vi "fo_SaveDatasetToFile.vi"(8 "error in (no error)":errorcluster, 9 "patientID":string="HALLO", 10 "Dataset index":i32, 11 "Results":refnum<k24>) -> (0 "error out":errorcluster)   [LabVIEW 2013, in "main.lvlib"]
uses:
  main.lvlib
  C:/Users/Simon/SkyDrive/LabView/2013/DM2020/bin/Dicom.dll
  bin/Dicom.dll
  Globals/DataPathGlobalVariable.vi
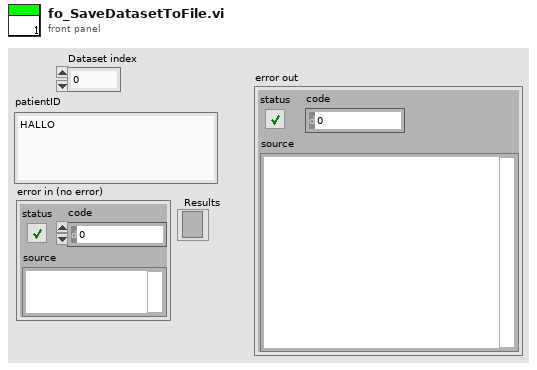
[diagram p1: front panel]
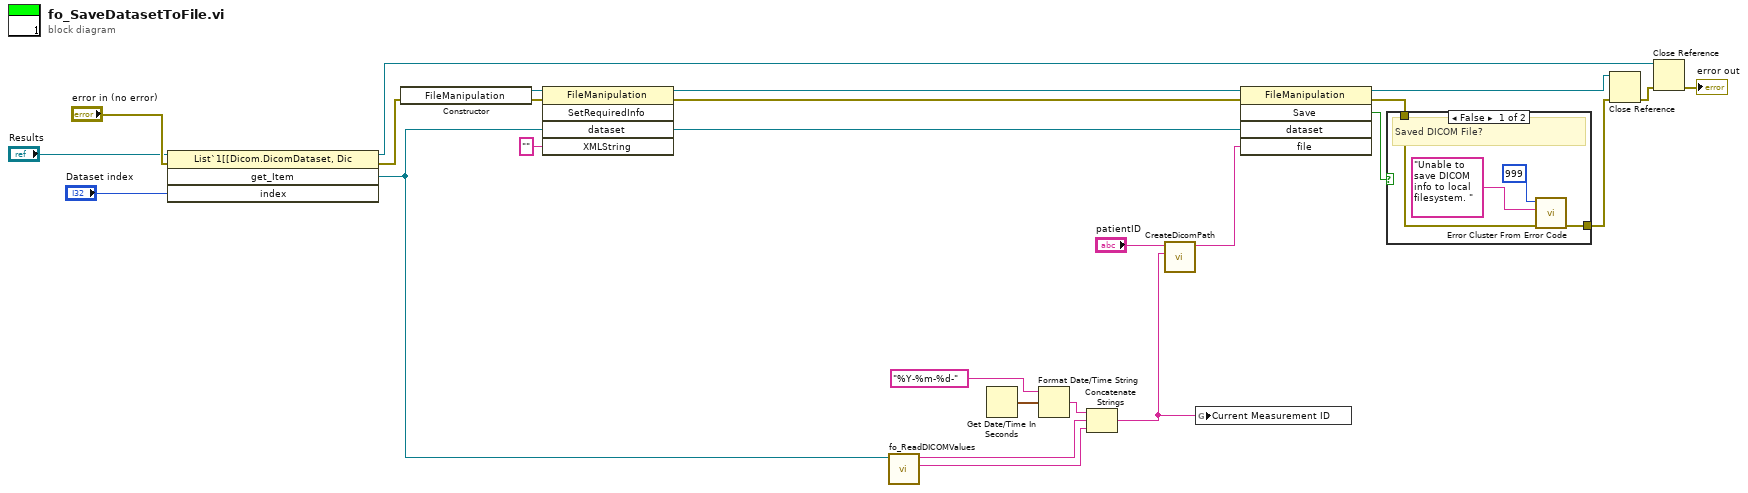
[diagram p0: block diagram]
diagram:
  n1 = invoke class="List`1[[Dicom.DicomDataset, Dic" method="get_Item"(reference="Results", error in="error in (no error)", "index"="Dataset index") -> (reference out=w16:refnum<k24>, error out=w15:errorcluster, "get_Item"=w5:refnum<k24>)  [unwired: 1 in, 1 out]
  n2 = constructor class="FileManipulation"(error in=w15) -> (reference out=w21:refnum<k24>, error out=w20:errorcluster)  [unwired: 2 in, 1 out]
  n3 = invoke class="FileManipulation" method="SetRequiredInfo"(reference=w21, error in=w20, "dataset"=w5, "XMLString"="") -> (reference out=w2:refnum<k24>, error out=w1:errorcluster)  [unwired: 1 in, 3 out]
  n4 = call "fo_ReadDICOMValues.vi"("dataset"=w5) -> ("study id"=w4:string, "accession number"=w3:string)  [unwired: 8 in, 1 out]
  n5 = Get Date/Time In Seconds() -> (seconds since 1Jan1904=w8:timestamp)
  n6 = Format Date/Time String(time format string (%c)="%Y-%m-%d-", seconds (now)=w8) -> (date/time string=w7:string)  [unwired: 1 in]
  n7 = Concatenate Strings(w7, w3, w4) -> (w6:string)
  n8 = call "CreateDicomPath.vi"("Measurement ID"=w6, "patientID"="patientID") -> ("String"=w22:string)  [unwired: 7 in, 2 out]
  n9 = global write "DataPathGlobalVariable.vi" "Current Measurement ID"(w6) -> ()
  n10 = invoke class="FileManipulation" method="Save"(reference=w2, error in=w1, "dataset"=w5, "file"=w22) -> (reference out=w24:refnum<k24>, error out=w12:errorcluster, "Save"=w11:bool)  [unwired: 1 in, 2 out]
  n11 = case shown="False" w11 {
    tunnel: w12 -> [w29 w30]
    tunnel: [w28 w30] -> w10
    frame False {
      # "Saved DICOM File?"
      n12 = call <vilib>:"Error Cluster From Error Code.vi"("error in (no error)"=w29, "error message (\"\")"="Unable to save DICOM info to local filesystem. " ("error message (\"\")"), "error code (0)"=999) -> ("error out"=w28:errorcluster)  [unwired: 6 in]
    }
    frame True {
    }
  }
  n13 = Close Reference(reference=w24, error in (no error)=w10) -> (error out=w23:errorcluster)
  n14 = Close Reference(reference=w16, error in (no error)=w23) -> (error out=→"error out":errorcluster)
